vi "Get File Content.vi"(8 "error in (no error)":errorcluster, 11 "read file in":refnum<class "read file.lvclass">) -> (0 "error out":errorcluster, 2 "file content":string, 3 "read file out":refnum<class "read file.lvclass">)   [LabVIEW 2017, in "read file.lvclass"]
doc: "Gets the file content with the file reference number from Read File.ctl. Use this VI as the VI under test for the Get File Content.lvtest test."
uses:
  read file.lvclass
  read file.lvclass/read file.ctl
panel:
  # "Overview: Gets the file content with the file reference number from Read File.ctl. Use this VI as the VI under test for the Get File Content.lvtest test."
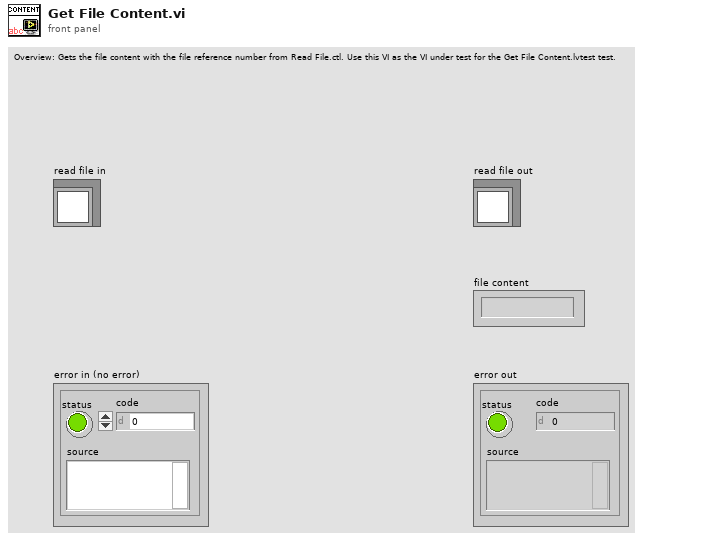
[diagram p1: front panel]
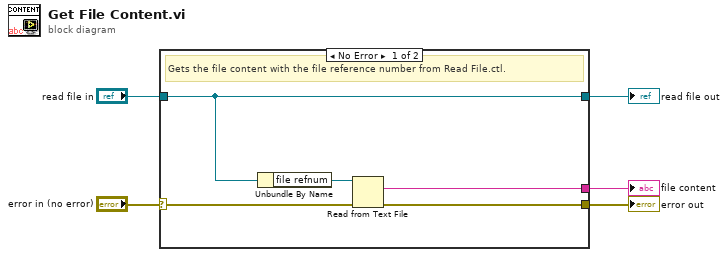
[diagram p0: block diagram]
diagram:
  n1 = case shown="No Error" "error in (no error)" {
    selector: "error in (no error)" -> [w9 w11]
    tunnel: [w8 w11] -> w4
    tunnel: [w10 w12] -> w2
    tunnel: "read file in" -> [w10 w12]
    tunnel: [w6 _] -> w1
    frame No Error {
      # "Gets the file content with the file reference number from Read File.ctl."
      n2 = Unbundle By Name(w10) -> ("file refnum"=w7:refnum<file>)
      n3 = Read from Text File(file (use dialog)=w7, error in=w9) -> (text=w6:string, error out=w8:errorcluster)  [unwired: 2 in, 2 out]
    }
    frame Error {
    }
  }
  "error out" <- w4
  "read file out" <- w2
  "file content" <- w1
